vi "Change State.vi"(8 "error in":errorcluster, 10 "New State":refnum<class "State Actor.lvclass">, 11 "State Actor in":refnum<class "State Actor.lvclass">) -> (0 "error out":errorcluster, 3 "State Actor out":refnum<class "State Actor.lvclass">)   [LabVIEW 2023, in "State Actor.lvlib" / "State Actor.lvclass"]
uses:
  Library/State Actor.lvclass
  C:/Users/Public/Documents/Development/builds/Engine/Actor Framework.lvlibp/1abvi3w/vi.lib/ActorFramework/Actor/Actor.lvclass
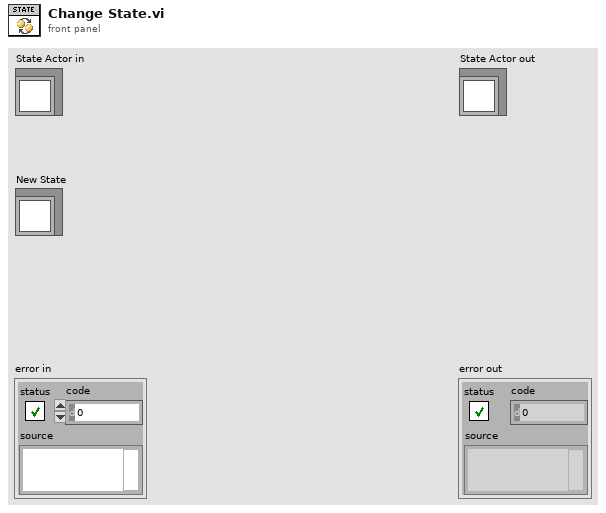
[diagram p1: front panel]
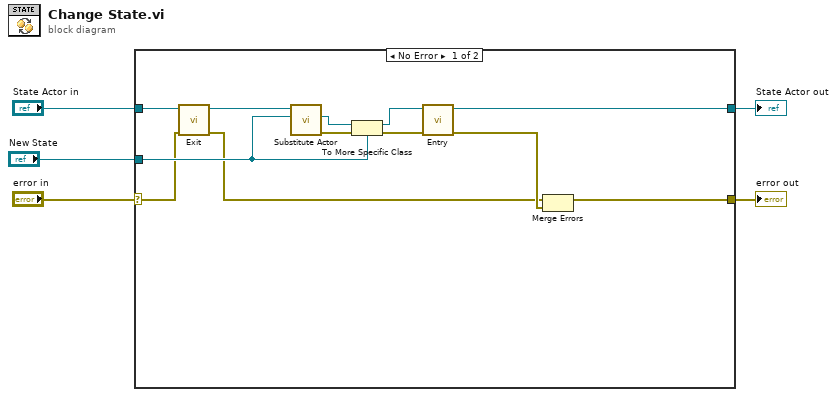
[diagram p0: block diagram]
diagram:
  n1 = case shown="No Error" "error in" {
    selector: "error in" -> [w7 w19]
    tunnel: [w9 w19] -> w4
    tunnel: [w11 w18] -> w2
    tunnel: "State Actor in" -> [w17 w18]
    tunnel: "New State" -> [w13 _]
    frame No Error {
      n2 = call-dynamic "Exit.vi"("error in (no error)"=w7, "State Actor in"=w17) -> ("error out"=w6:errorcluster, "State Actor out"=w16:refnum<class "State Actor.lvclass">)  [unwired: 8 in]
      n3 = call-dynamic "Substitute Actor.vi"("Substitute Actor in"=w13, "Current Panel Actor"=w16) -> ("error out"=w15:errorcluster, "Substitute Actor out"=w14:refnum<class "Actor.lvclass">)  [unwired: 8 in]
      n4 = To More Specific Class(target class=w13, reference=w14, error in=w15) -> (specific class reference=w12:refnum<class "State Actor.lvclass">, error out=w10:errorcluster)
      n5 = call-dynamic "Entry.vi"("error in (no error)"=w10, "State Actor in"=w12) -> ("error out"=w8:errorcluster, "State Actor out"=w11:refnum<class "State Actor.lvclass">)  [unwired: 8 in]
      n6 = Merge Errors(w6, w8) -> (w9:errorcluster)
    }
    frame Error {
    }
  }
  "error out" <- w4
  "State Actor out" <- w2
